vi "读取字节数组.vi"(8 "error in (no error)":errorcluster caption="错误输入（无错误）", 10 "count":i32, 11 "串口 输入":refnum<class "串口.lvclass"> caption="DNL_LabVIEW Object in") -> (0 "error out":errorcluster caption="错误输出", 1 "Read":i32, 2 "Bytes":u8[](array[numeric]), 3 "串口 输出":refnum<class "串口.lvclass"> caption="DNL_LabVIEW Object out")   [LabVIEW 2012, in "串口.lvclass"]
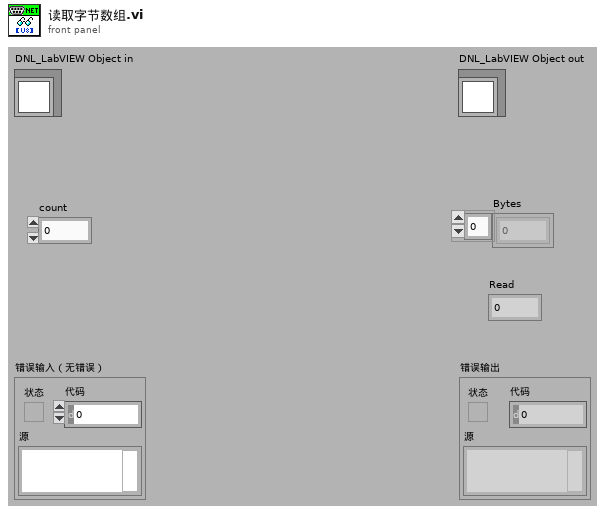
[diagram p1: front panel]
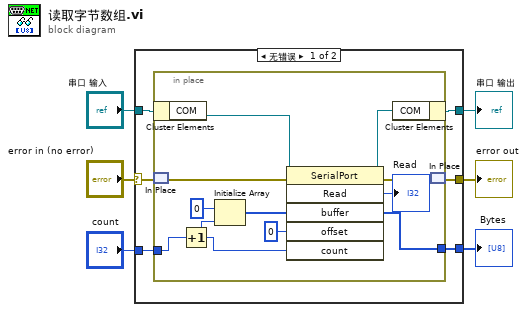
[diagram p0: block diagram]
diagram:
  n1 = case shown="无错误" "error in (no error)" {
    selector: "error in (no error)" -> [w11 w25]
    tunnel: [w10 w25] -> w5
    tunnel: [w7 w24] -> w3
    tunnel: "串口 输入" -> [w12 w24]
    tunnel: "count" -> [w9 _]
    tunnel: [w8 _] -> w1
    frame No Error {
      n2 = in-place {
        in-place-border: w9 -> [w14]
        in-place-border: [w17] -> w8
        n3 = in-place-cluster #1(w12) -> ("COM"=w23:refnum<k24>)
        n4 = in-place-match #2(w11) -> (w21:errorcluster)
        n5 = Increment(x=w14) -> (x+1=w13:i32)
        n6 = Initialize Array(u8 0 ("元素"), w13) -> (w18:u8[])
        n7 = invoke class="SerialPort" method="Read"(reference=w23, error in=w21, "buffer"=w18, "offset"=0, "count"=w13) -> (reference out=w22:refnum<k24>, error out=w20:errorcluster, "Read"=→"Read":i32, "buffer"=w17:u8[])  [unwired: 1 in, 2 out]
        n8 = in-place-cluster #1("COM"=w22) -> (w7:refnum<class "串口.lvclass">)
        n9 = in-place-match #2(w20) -> (w10:errorcluster)
      }
    }
    frame Error {
    }
  }
  "error out" <- w5
  "串口 输出" <- w3
  "Bytes" <- w1
